vi "SetCoarse.vi"(8 "error in":T2, 11 "Coarse Input":T1 {"Amplitude" format="%.0f V"; "Frequency" format="%.0f Hz"}) -> (0 "error out":T2, 3 "coarse output cluster":T1 {"Amplitude" format="%.0f V"; "Frequency" format="%.0f Hz"})   [LabVIEW 2016]
doc: "Prepares an axis for coarse movement. The number of the axis is a required input and restricted from 0 to 2 corresponding to axis 1 to axis 3. The frequency should be given in hertz and may range from 1 to 8000Hz. Whereas the amplitude is given in volt and is restricted to a range from 0 to 70V.\nBy passing -Inf (float) or -2147483648 (integer) as input values, the corresponding parameter(s) will be read out."
uses:
  Controls/Error_Out.ctl
  Files_ASC500/DLL/ASC500_RemoteControlV27.dll
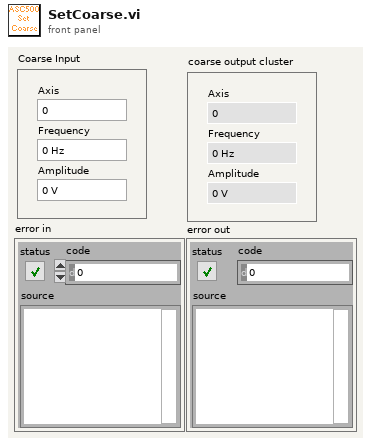
[diagram p1: front panel]
types:
  T1 = cluster{"Axis":i32, "Frequency":i32, "Amplitude":i32}
  T2 = typedef "Error_Out.ctl" = errorcluster
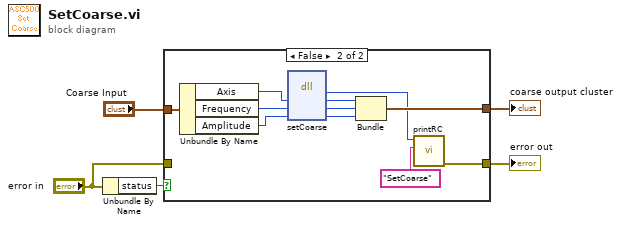
[diagram p0: block diagram]
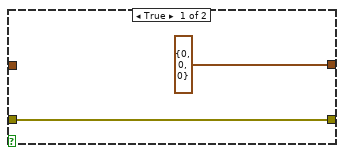
[diagram p2: hidden frame]
diagram:
  n1 = Unbundle By Name("error in") -> ("status"=w5:bool)
  n2 = case shown="False" w5 {
    tunnel: [w6 w14] -> w4
    tunnel: [T1 {"Axis"=0, "Frequency"=0, "Amplitude"=0} w15] -> w3
    tunnel: "error in" -> [w6 _]
    tunnel: "Coarse Input" -> [_ w11]
    frame True {
    }
    frame False {
      n3 = Unbundle By Name(w11) -> ("Axis"=w10:i32, "Frequency"=w9:i32, "Amplitude"=w8:i32)
      n4 = dll-call lib="G:/SCMOperations/Share/ELE/Produkt Information/ASC500/04 Remote Control/02 development versions/2018Nov06/Files_ASC500/DLL/ASC500_RemoteControlV27.dll" fn="setCoarse"("Axis"=w10, "Frequency"=w9, "Amplitude"=w8) -> ("return type"=w13:i32, "Axis"=w18:i32, "Frequency"=w17:i32, "Amplitude"=w16:i32)  [unwired: 3 in, 2 out]
      n5 = Bundle("Axis"=w18, "Frequency"=w17, "Amplitude"=w16) -> (w15:T1)  [unwired: 1 in]
      n6 = call "printRC.vi"("additional information"="SetCoarse", "RC"=w13) -> ("error out"=w14:T2)  [unwired: 9 in]
    }
  }
  "error out" <- w4
  "coarse output cluster" <- w3
